vi "Stop Sequence.vi"(8 "error in (no error)":errorcluster, 11 "Connection Data In":T1) -> (0 "error out":errorcluster, 3 "Connection Data Out":T1)   [LabVIEW 2014, in "MSX-E3701_dll.lvlib"]
doc: "Detiene la Adquisición del modo Séquence."
uses:
  MSX-E3701_dll.lvlib
  Typedef/Connection Data.ctl
  E:/Repositorio Magnis/INF002/v0/Modules/HAL/Drivers/Sync/ADDI-DATA MSX-E3701/API/MX370x.dll
  MX370x.dll
  E:/Repositorio Magnis/INF002/v0/Modules/HAL/Drivers/Sync/ADDI-DATA MSX-E3701/API/MXCommon.dll
  MXCommon.dll
panel:
  out "ESTATUS DE STOP DEL SISTEMA":string="Success"
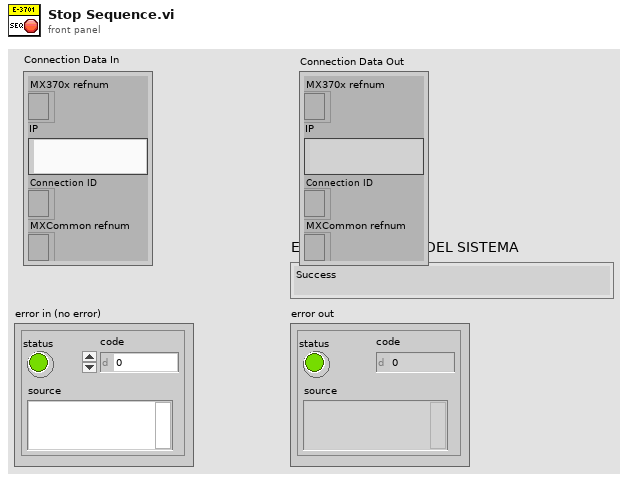
[diagram p1: front panel]
types:
  T1 = typedef "MSX-E3701_dll.lvlib/Connection Data.ctl" = cluster{"MX370x refnum":refnum<k24>, "IP":string, "Connection ID ":refnum<k5>, "MXCommon refnum":refnum<k24>}
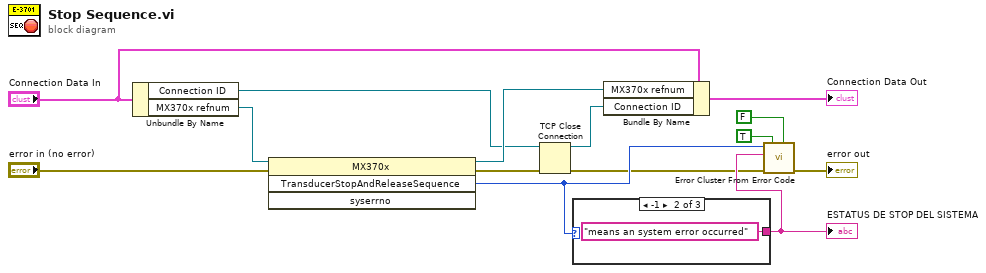
[diagram p0: block diagram]
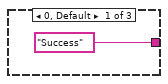
[diagram p2: hidden frame]
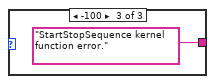
[diagram p3: hidden frame]
diagram:
  n1 = Unbundle By Name("Connection Data In") -> ("Connection ID"=w2:refnum<k5>, "MX370x refnum"=w5:refnum<k24>)
  n2 = invoke class="MX370x" method="TransducerStopAndReleaseSequence"(reference=w5, error in="error in (no error)") -> (reference out=w8:refnum<k24>, error out=w4:errorcluster, "TransducerStopAndReleaseSequence"=w7:i32)  [unwired: 2 in, 1 out]
  n3 = TCP Close Connection(connection ID=w2, error in (no error)=w4) -> (connection ID out=w1:refnum<k5>, error out=w3:errorcluster)  [unwired: 1 in]
  n4 = case shown="-1" w7 {
    tunnel: ["Success" "means an system error occurred" "StartStopSequence kernel function error."] -> w11
    frame 0, Default {
    }
    frame -1 {
    }
    frame -100 {
    }
  }
  "ESTATUS DE STOP DEL SISTEMA" <- w11
  n5 = Bundle By Name(cluster="Connection Data In", "MX370x refnum"=w8, "Connection ID"=w1) -> (→"Connection Data Out":T1)
  n6 = call <vilib>:"Error Cluster From Error Code.vi"("is warning? (False)"=FALSE, "show call chain? (False)"=TRUE, "error in (no error)"=w3, "error message (\"\")"=w11, "error code (0)"=w7) -> ("error out"=→"error out":errorcluster)  [unwired: 4 in]
